vi "AVI_Test.vi"() -> ()   [LabVIEW 2009]
uses:
  <vilib>/imath/engines/lvmath2/RunTimeEngine/ErrorHandling/NIMS_Finalize Error.vi
  <vilib>/imath/engines/lvmath2/RunTimeEngine/Parser/MC_Version.vi
  <vilib>/imath/engines/lvmath2/RunTimeEngine/NodeEndStatement/NIMS_NodeEndStatement_Output.vi
  <instcachedir>/0/NIMS_NodeEndStatement_Output_B70DDD75627E4997AAE11E9955EDAA25.lvgen/NIMS_NodeEndStatement_Output_B70DDD75627E4997AAE11E9955EDAA25_001.vi
  <vilib>/imath/engines/lvmath/Functions/Error Handling/MergeErrorsWrapper.vi
  <vilib>/vision/NI_Vision_Development_Module.lvlib
panel:
  out "rectangle":i32[](array[numeric])=[103, 210, 569, 367]
  in  "Change ROI":bool
  out "ROI":T1(plugin-control)
  in  "Slide":u32(slide)=143 scale=0.0..8620.0
  in  "stop":bool
  out "Image":T1(plugin-control)
  out "Start Time":u32=3771410
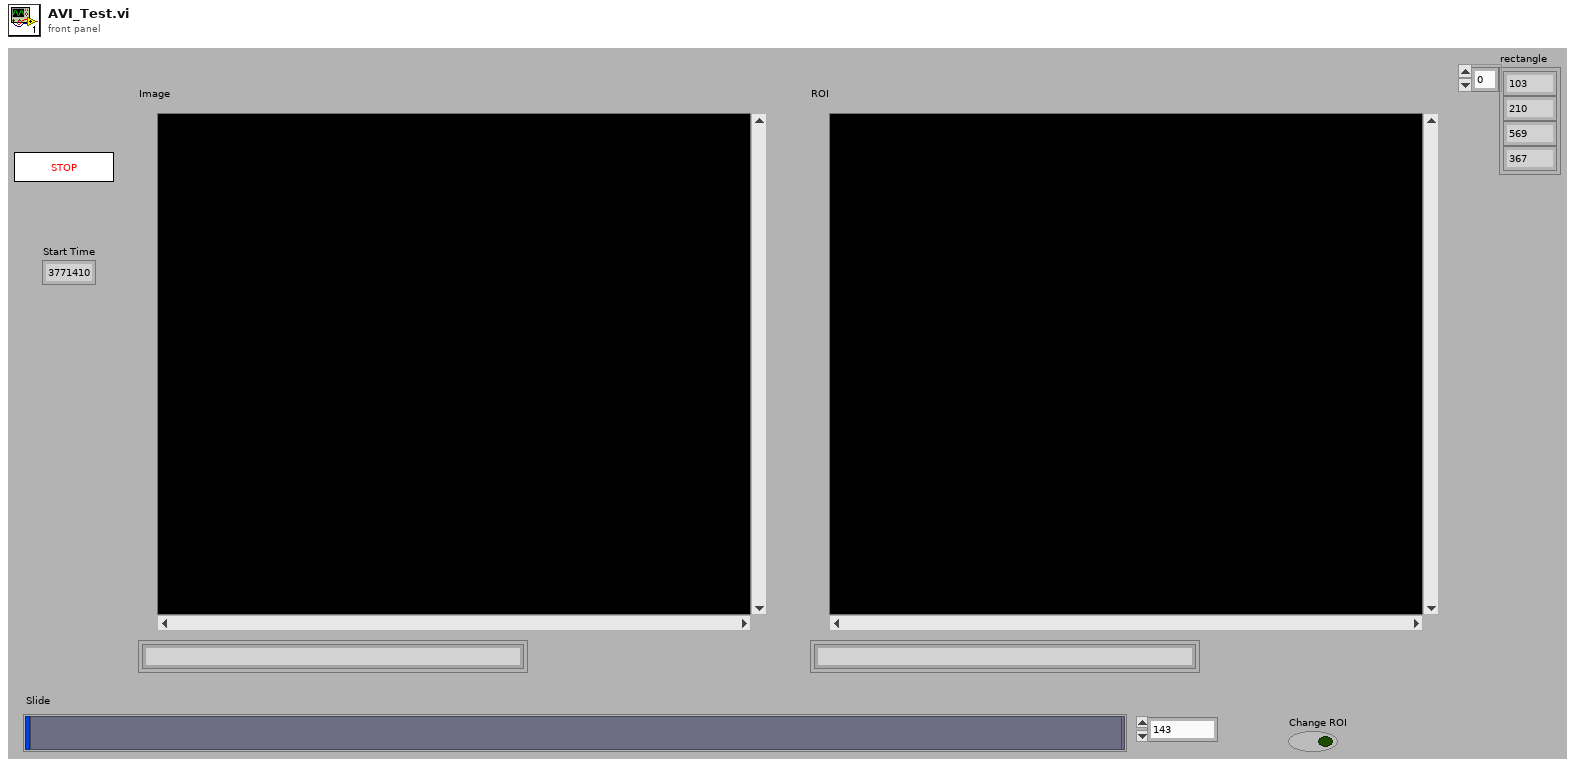
[diagram p1: front panel]
types:
  T1 = typedef "IMAQ Image.ctl" = refnum<image>
  T2 = typedef "Image Type" = u32
  T3 = enum32{"existing file", "new file", "new or existing file", "existing dir", "new dir", "new or existing dir", "existing file (use LLBs)", "new file (use LLBs)", "new or existing file (use LLBs)", "new or existing file or directory (use LLBs)"}
  T4 = typedef "AviRefnum.ctl" = refnum<k1>
  T5 = cluster{"width":u32, "height":u32, "framesPerSecond":u32, "compressionFilter":string, "hasData":bool}
  T6 = typedef "IMAQ Rectangle" = cluster{"Left":i32, "Top":i32, "Right":i32, "Bottom":i32, "Rotation":dbl}
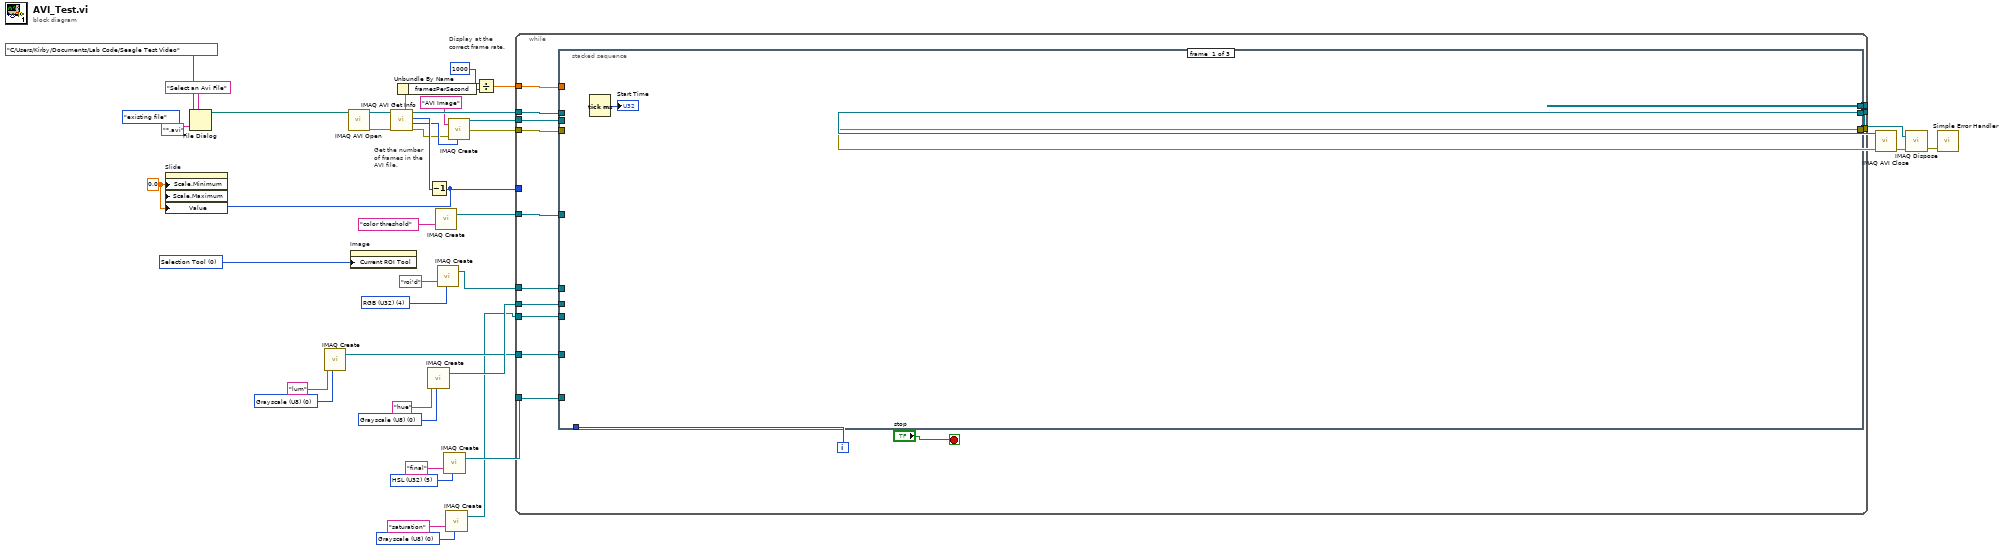
[diagram p0: block diagram]
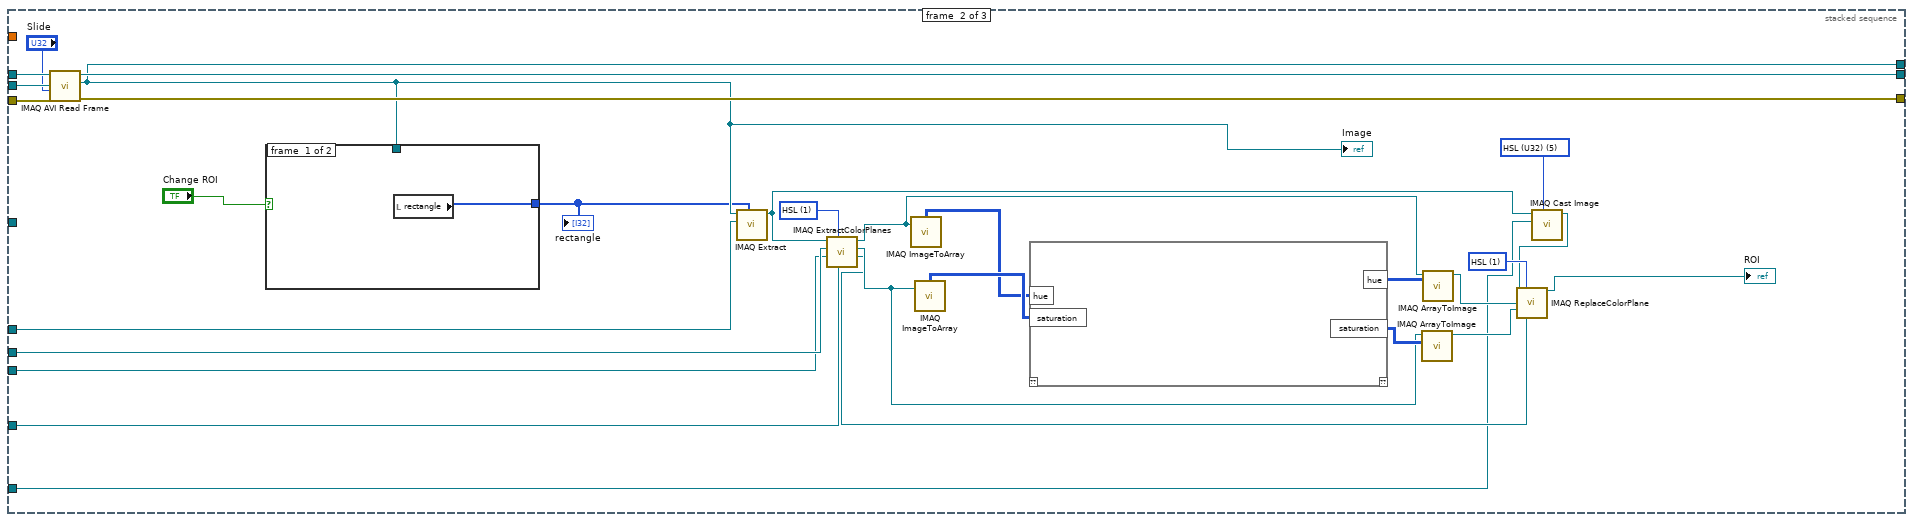
[diagram p2: hidden frame]
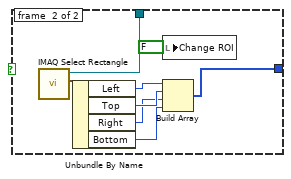
[diagram p3: hidden frame]
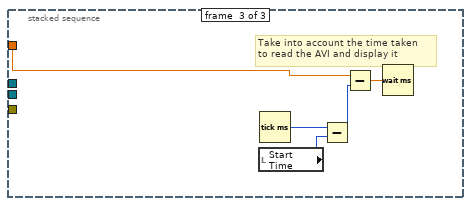
[diagram p4: hidden frame]
diagram:
  w4 = T2 0 items=["Grayscale (U8)", "Grayscale (I16)", "Grayscale (SGL)", "Complex (CSG)", "RGB (U32)", "HSL (U32)", "RGB (U64)", "Grayscale (U16)"] ("Image Type")
  w6 = T2 5 items=["Grayscale (U8)", "Grayscale (I16)", "Grayscale (SGL)", "Complex (CSG)", "RGB (U32)", "HSL (U32)", "RGB (U64)", "Grayscale (U16)"] ("Image Type")
  w8 = u32 0 items=["Zoom Tool"=8, "Selection Tool"=0, "Pan Tool"=9, "Point Tool"=1, "Line Tool"=2, "Rectangle Tool"=3, "Rotated Rectangle Tool"=12, "Polyline Tool"=10, "Polygon Tool"=5, "Freehand Tool"=11, "Closed Freehand Tool"=6, "Ellipse Tool"=4, "Annulus Tool"=7] ("Current ROI Tool")
  w9 = T2 4 items=["Grayscale (U8)", "Grayscale (I16)", "Grayscale (SGL)", "Complex (CSG)", "RGB (U32)", "HSL (U32)", "RGB (U64)", "Grayscale (U16)"] ("Image Type")
  w11 = T2 0 items=["Grayscale (U8)", "Grayscale (I16)", "Grayscale (SGL)", "Complex (CSG)", "RGB (U32)", "HSL (U32)", "RGB (U64)", "Grayscale (U16)"] ("Image Type")
  w12 = T2 0 items=["Grayscale (U8)", "Grayscale (I16)", "Grayscale (SGL)", "Complex (CSG)", "RGB (U32)", "HSL (U32)", "RGB (U64)", "Grayscale (U16)"] ("Image Type")
  w13 = 0.0 ("Scale.Range:Minimum")
  (unwired) T3."existing file" ("select mode (2)")
  # "Display at the \ncorrect frame rate."
  # "Get the number\nof frames in the\nAVI file."
  n1 = File Dialog(6:"*.avi" ("pattern"), 7:"Select an Avi File" ("prompt"), 11:path "C:/Users/Kirby/Documents/Lab Code/Seagle Test Video" ("start path")) -> (3:w22:path)  [unwired: 1 in, 6 out]
  n2 = call "IMAQ Create"("Image Name"="lum", "Image Type"=w4) -> ("New Image"=w2:T1)  [unwired: 3 in, 1 out]
  n3 = call "IMAQ AVI Open"("AVI Path"=w22) -> ("error out"=w30:errorcluster, "Avi Refnum"=w31:T4)  [unwired: 1 in, 8 out]
  n4 = property on="Image" class="ImageControl"("Current ROI Tool"=w8) -> ()  [unwired: 2 in, 2 out]
  n5 = call "IMAQ AVI Get Info"("error in (no error)"=w30, "Avi Refnum"=w31) -> ("error out"=w35:errorcluster, "Image Type"=w41:T2, "Number of Frames"=w42:u32, "Avi Refnum (duplicate)"=w38:T4, "Frame Data"=w26:T5)  [unwired: 5 out]
  n6 = Unbundle By Name(w26) -> ("framesPerSecond"=w29:u32)
  n7 = call "IMAQ Create"("Image Name"="hue", "Image Type"=w12) -> ("New Image"=w15:T1)  [unwired: 3 in, 1 out]
  n8 = Decrement(x=w42) -> (x-1=w14:u32)
  n9 = property on="Slide" class="Slide (strict)"("Scale.Minimum"=w13, "Scale.Maximum"=w14, "Value"=w13) -> ()  [unwired: 2 in, 2 out]
  n10 = call "IMAQ Create"("Image Name"="color threshold") -> ("New Image"=w20:T1)  [unwired: 4 in, 1 out]
  n11 = call "IMAQ Create"("Image Name"="roi'd", "Image Type"=w9) -> ("New Image"=w17:T1)  [unwired: 3 in, 1 out]
  n12 = call "IMAQ Create"("Image Name"="final", "Image Type"=w6) -> ("New Image"=w5:T1)  [unwired: 3 in, 1 out]
  n13 = call "IMAQ Create"("Image Name"="saturation", "Image Type"=w11) -> ("New Image"=w1:T1)  [unwired: 3 in, 1 out]
  n14 = call "IMAQ Create"("Image Name"="AVI Image", "Image Type"=w41, "error in (no error)"=w35) -> ("New Image"=w37:T1, "error out"=w36:errorcluster)  [unwired: 1 in, 1 out]
  n15 = Divide(x=1000, y=w29) -> (x/y=w28:dbl)
  n16 = while {
    tunnel: w37 -> [w54]
    tunnel: [w55] -> w33
    tunnel: [w50] -> w32
    tunnel: w28 -> [w51]
    tunnel: w36 -> [w56]
    tunnel: w38 -> [w57]
    tunnel: [w53] -> w40
    tunnel: w14 -> [_]
    tunnel: w20 -> [w49]
    tunnel: w17 -> [w48]
    tunnel: w15 -> [w47]
    tunnel: w1 -> [w46]
    tunnel: w5 -> [w44]
    tunnel: w2 -> [w43]
    i -> [w52]
    stop <- "stop" stop-if-true
    n17 = stacked-sequence {
      tunnel: w57 -> [_ w87 _]
      tunnel: w56 -> [_ w86 _]
      tunnel: [_ w85 _] -> w55
      tunnel: w54 -> [_ w84 _]
      tunnel: [_ w80 _] -> w53
      tunnel: w52 -> [_ _ _]
      tunnel: w51 -> [_ _ w114]
      tunnel: [_ w83 _] -> w50
      tunnel: w49 -> [_ _ _]
      tunnel: w48 -> [_ w78 _]
      tunnel: w47 -> [_ w68 _]
      tunnel: w46 -> [_ w67 _]
      tunnel: w44 -> [_ w61 _]
      tunnel: w43 -> [_ w66 _]
      frame #0 {
        n18 = Tick Count (ms)() -> (millisecond timer value=→"Start Time":u32)
      }
      frame #1 {
        w60 = T2 5 items=["Grayscale (U8)", "Grayscale (I16)", "Grayscale (SGL)", "Complex (CSG)", "RGB (U32)", "HSL (U32)", "RGB (U64)", "Grayscale (U16)"] ("Image Type")
        w69 = u16 1 items=["RGB", "HSL", "HSV", "HSI"] ("Color Mode")
        w75 = u16 1 items=["RGB", "HSL", "HSV", "HSI"] ("Color Mode")
        n19 = call "IMAQ AVI Read Frame"("error in (no error)"=w86, "Frame Number"="Slide", "Image"=w84, "Avi Refnum"=w87) -> ("error out"=w83:errorcluster, "Image Out"=w80:T1, "Avi Refnum (duplicate)"=w85:T4)  [unwired: 1 in, 4 out]
        "Image" <- w80
        n20 = case shown="False" "Change ROI" {
          tunnel: w80 -> [_ w113]
          tunnel: [w105 w106] -> w79
          frame #0 {
            n21 = local read "rectangle"() -> (w105:i32[])
          }
          frame #1 {
            n22 = call "IMAQ Select Rectangle"("Image In"=w113) -> ("Rectangle"=w112:T6)  [unwired: 7 in, 3 out]
            n23 = Unbundle By Name(w112) -> ("Left"=w110:i32, "Top"=w109:i32, "Right"=w108:i32, "Bottom"=w107:i32)
            n24 = local write "Change ROI"(FALSE ("Boolean")) -> ()
            n25 = Build Array(w110, w109, w108, w107) -> (w106:i32[])
          }
        }
        "rectangle" <- w79
        n26 = call "IMAQ Extract"("Optional Rectangle"=w79, "Image Dst"=w78, "Image Src"=w80) -> ("Image Dst Out"=w62:T1)  [unwired: 7 in, 1 out]
        n27 = call "IMAQ ExtractColorPlanes"("Blue or Luma or Val or Inten Plane"=w66, "Color Mode"=w69, "Green or Sat Plane"=w67, "Red or Hue Plane"=w68, "Image Src"=w62) -> ("Blue or Luma or Val or Inten Plane out"=w63:T1, "Green or Sat Plane out"=w64:T1, "Red or Hue Plane out"=w65:T1)  [unwired: 3 in, 1 out]
        n28 = call "IMAQ ImageToArray"("Image"=w65) -> ("Image Pixels (U8)"=w76:u8[][])  [unwired: 3 in, 4 out]
        n29 = call "IMAQ ImageToArray"("Image"=w64) -> ("Image Pixels (U8)"=w77:u8[][])  [unwired: 3 in, 4 out]
        n30 = mathscript code="1"("hue"=w76, "saturation"=w77) -> ("hue"=w73:u8[][], "saturation"=w74:u8[][])  [unwired: 1 in, 1 out]
        n31 = call "IMAQ ArrayToImage"("Image Pixels (U8)"=w74, "Image"=w64) -> ("Image Out"=w71:T1)  [unwired: 8 in, 1 out]
        n32 = call "IMAQ ArrayToImage"("Image Pixels (U8)"=w73, "Image"=w65) -> ("Image Out"=w72:T1)  [unwired: 8 in, 1 out]
        n33 = call "IMAQ Cast Image"("Image Type"=w60, "Image Dst"=w61, "Image Src"=w62) -> ("Image Dst Out"=w59:T1)  [unwired: 7 in, 1 out]
        n34 = call "IMAQ ReplaceColorPlane"("Image Src"=w59, "Color Mode"=w75, "Red or Hue Plane"=w72, "Green or Sat Plane"=w71, "Blue or Luma or Val or Inten Plane"=w63) -> ("Image Dst Out"=→"ROI":T1)  [unwired: 9 in, 1 out]
      }
      frame #2 {
        # "Take into account the time taken \nto read the AVI and display it"
        n35 = local read "Start Time"() -> (w117:u32)
        n36 = Tick Count (ms)() -> (millisecond timer value=w118:u32)
        n37 = Subtract(x=w118, y=w117) -> (x-y=w116:u32)
        n38 = Subtract(x=w114, y=w116) -> (x-y=w115:dbl)
        n39 = Wait (ms)(milliseconds to wait=w115) -> ()  [unwired: 1 out]
      }
    }
  }
  n40 = call "IMAQ AVI Close"("error in (no error)"=w32, "Avi Refnum"=w33) -> ("error out"=w39:errorcluster)  [unwired: 9 out]
  n41 = call "IMAQ Dispose"("Image"=w40, "error in (no error)"=w39) -> ("error out"=w25:errorcluster)  [unwired: 1 in, 3 out]
  n42 = call <vilib>:"Simple Error Handler.vi"("error in (no error)"=w25) -> ()  [unwired: 1 in, 8 out]
